vi "BuildHdrFilePath.vi"(2 "error in":errorcluster, 3 "Destination:":path) -> (0 "error in (no error)":errorcluster, 1 "configuration file path":path)   [LabVIEW 2009]
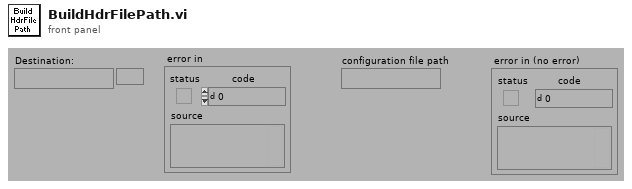
[diagram p1: front panel]
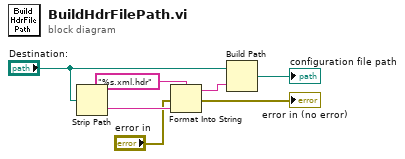
[diagram p0: block diagram]
diagram:
  n1 = Strip Path(path="Destination:") -> (name=w7:string)  [unwired: 1 out]
  n2 = Format Into String(format string="%s.xml.hdr", error in="error in", w7) -> (resulting string=w3:string, error out=→"error in (no error)":errorcluster)  [unwired: 1 in]
  n3 = Build Path(base path="Destination:", name or relative path=w3) -> (appended path=→"configuration file path":path)
